vi "ArrayLastValue.vi"(1 "Array In":dbl[](array[numeric])) -> (0 "Last value":dbl)   [LabVIEW 2014]
doc: "André Romero - 2017\nandretec@ifsc.usp.br"
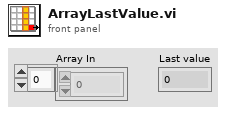
[diagram p1: front panel]
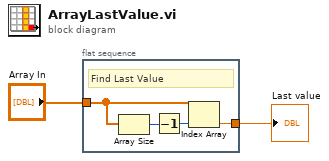
[diagram p0: block diagram]
diagram:
  n1 = flat-sequence {
    tunnel: [w4] -> w2
    tunnel: "Array In" -> [w3]
    frame #0 {
      # "Find Last Value"
      n2 = Array Size(array=w3) -> (size(s)=w6:i32)
      n3 = Decrement(x=w6) -> (x-1=w5:i32)
      n4 = Index Array(array=w3, index=w5) -> (element=w4:dbl)
    }
  }
  "Last value" <- w2
